vi "循环扫描数据分离.vi"(11 "数据":dbl[][](array[numeric])) -> (1 "RE开始":dbl, 2 "RESET":dbl[][](array[numeric]), 3 "SET":dbl[][](array[numeric]))   [LabVIEW 2021]
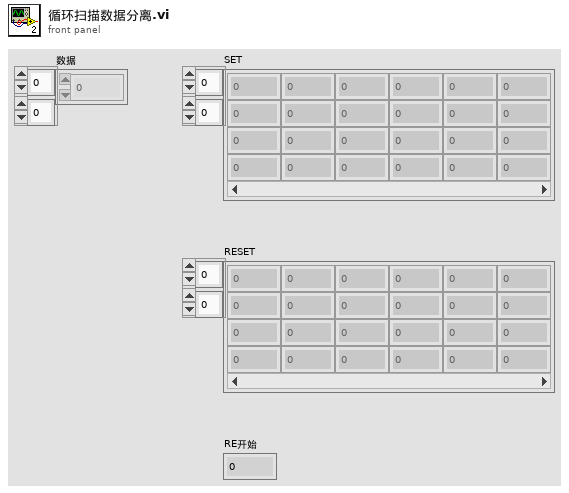
[diagram p1: front panel]
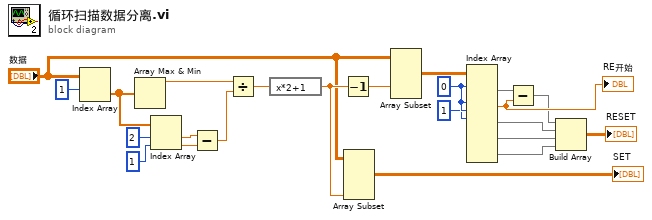
[diagram p0: block diagram]
diagram:
  w10 = 0 ("索引 (行)")
  n1 = Index Array(array="数据", index (row)=1 ("索引 (行)")) -> (element=w23:dbl[])  [unwired: 1 in]
  n2 = Array Max & Min(array=w23) -> (max value=w18:dbl)  [unwired: 3 out]
  n3 = Index Array(array=w23, index #1=2 ("索引"), index #2=1 ("索引")) -> (element #1=w20:dbl, element #2=w19:dbl)
  n4 = Subtract(x=w20, y=w19) -> (x-y=w17:dbl)
  n5 = Divide(x=w18, y=w17) -> (x/y=w14:dbl)
  n6 = expression code="x*2+1"(w14) -> (w13:dbl)
  n7 = Decrement(x=w13) -> (x-1=w12:dbl)
  n8 = Array Subset(array="数据", length (col)=w13) -> (→"SET":dbl[][])  [unwired: 3 in]
  n9 = Array Subset(array="数据", index (col)=w12) -> (w11:dbl[][])  [unwired: 3 in]
  n10 = Index Array(array=w11, index (row) #1=w10, index (row) #2=w10, index (col) #2=w10, index (row) #3=1 ("索引 (行)")) -> (element #1=w9:dbl[], element #2=w8:dbl, element #3=w5:dbl[], element #4=w4:dbl[], element #5=w3:dbl[])  [unwired: 6 in]
  "RE开始" <- w8
  n11 = Subtract(x=w9, y=w8) -> (x-y=w6:dbl[])
  n12 = Build Array(w6, w5, w4, w3) -> (→"RESET":dbl[][])
